vi "Complex absolute value.vi"(8 "Im":fxp<+/-,22,22>, 11 "Re":fxp<+/-,22,22>) -> (2 "Square Absolute Value":fxp<+,44,44>)   [LabVIEW 2014]
doc: "This subVI computes the square absolute value of a complex number"
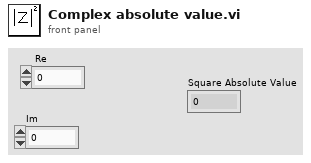
[diagram p1: front panel]
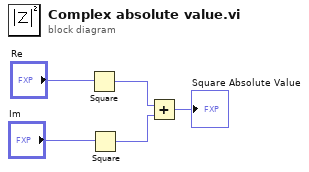
[diagram p0: block diagram]
diagram:
  n1 = Square(x="Re") -> (x^2=w3:fxp<+,43,43>)
  n2 = Square(x="Im") -> (x^2=w2:fxp<+,43,43>)
  n3 = Add(x=w3, y=w2) -> (x+y=→"Square Absolute Value":fxp<+,44,44>)
